vi "VarShareVI.vi"() -> ()   [LabVIEW 2011]
panel:
  in  "DummyVar":dbl(slide) scale=0.0..10.0
  in  "stop":bool
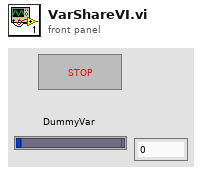
[diagram p1: front panel]
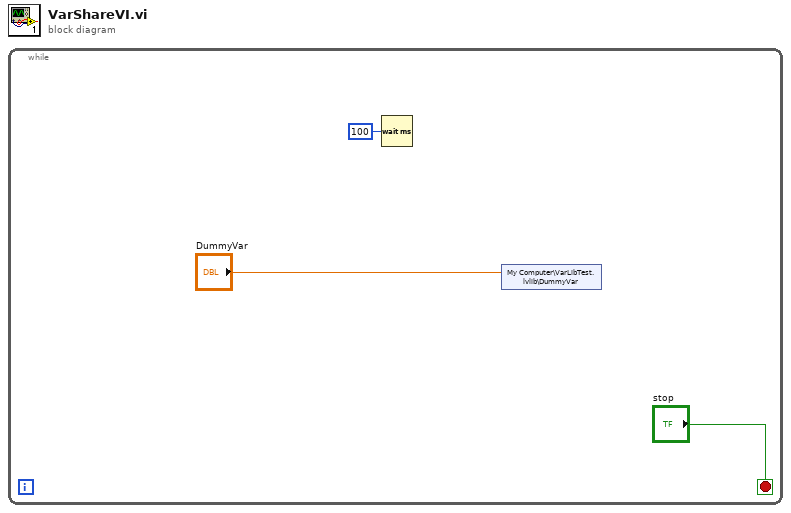
[diagram p0: block diagram]
diagram:
  n1 = while {
    stop <- "stop" stop-if-true
    n2 = Wait (ms)(milliseconds to wait=u32 100) -> ()  [unwired: 1 out]
    n3 = shared-variable "My Computer\\VarLibTest.lvlib\\DummyVar"("DummyVar") -> ()  [unwired: 1 in, 1 out]
  }
